vi "LanguageList.vi"(10 "LanguageList":string) -> (0 "Fehler (Ausgang)":errorcluster, 1 "Sprachen Anzahl":i32, 2 "Sprache full":T2 caption="Please select a language:" items=["Deutsch", "English", "Français", "Italiano", "Castellano", "Polski"], 3 "Strings und Werte []":T1, 4 "FullLanguageList":u16[](array[numeric]), 5 "FullLanguageList":string)   [LabVIEW 2015, in "Sprachverwaltung.lvlib"]
doc: "Sprachauswahl für Auswahlfeld nach einer Liste (Indexzahlen getrennt mit Komma) aus der Geasmtsprachliste.\nGibt die Geasmtsprachliste, Anzahl der Sprachen, Indexliste aller Spreachen und die Sprachauswahl zurück.\nRIW 2019-11-29 (Black Friday)s"
uses:
  Sprachverwaltung.lvlib
  Allgemein/Sprachauswahl native.ctl
  <vilib>/Utility/miscctls.llb/LVStringsAndValuesArrayTypeDef_U16.ctl
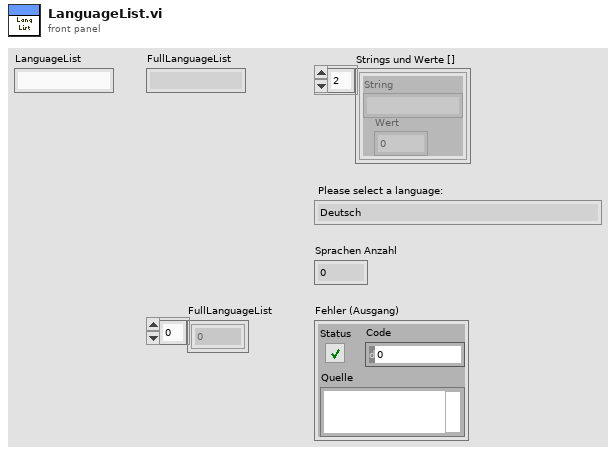
[diagram p1: front panel]
types:
  T1 = typedef "LVStringsAndValuesArrayTypeDef_U16.ctl" = cluster{"String":string, "Value":u16}[]
  T2 = typedef "Sprachverwaltung.lvlib/Sprachauswahl native.ctl" = u16
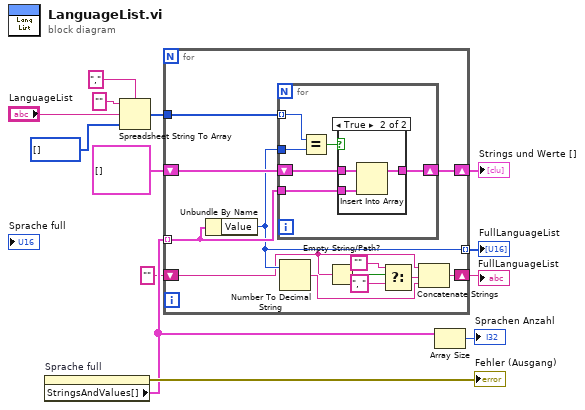
[diagram p0: block diagram]
diagram:
  n1 = property on="Sprache full" class="Ring (strikt)"() -> (error out=→"Fehler (Ausgang)":errorcluster, "StringsAndValues[]"=w5:T1)  [unwired: 2 in, 1 out]
  n2 = Spreadsheet String To Array(delimiter (Tab)="," ("Trennzeichen (Tabulator)"), format string="" ("Format-String"), spreadsheet string="LanguageList", array type (2D Dbl)=u16[] []) -> (array=w11:u16[])
  n3 = for {
    tunnel: w11 -> [w25]
    tunnel: w5 -> [w22] mode=indexing
    shift-right: [w24] -> w6
    shift-left: T1 [] ("Strings und Werte []") -> [w23]
    tunnel: [w21] -> w3 mode=indexing
    shift-right: [w20] -> w2
    shift-left: "" -> [w18]
    n4 = Unbundle By Name(w22) -> ("Value"=w21:u16)
    n5 = for {
      tunnel: w21 -> [w26]
      tunnel: w25 -> [w31] mode=indexing
      tunnel: w22 -> [w29]
      shift-right: [w28] -> w24
      shift-left: w23 -> [w27]
      n6 = Equal?(x=w31, y=w26) -> (x = y?=w30:bool)
      n7 = case shown="True" w30 {
        tunnel: w27 -> [w32 w35]
        tunnel: [w32 w34] -> w28
        tunnel: w29 -> [_ w33]
        frame False {
        }
        frame True {
          n8 = Insert Into Array(array=w35, new element=w33) -> (w34:T1)  [unwired: 1 in]
        }
      }
    }
    n9 = Number To Decimal String(number=w21) -> (decimal integer string=w19:string)  [unwired: 1 in]
    n10 = Empty String/Path?(string/path=w18) -> (empty?=w17:bool)
    n11 = Select(t="", s=w17, f=", " ("String")) -> (s? t:f=w15:string)
    n12 = Concatenate Strings(w18, w15, w19) -> (w20:string)
  }
  "Strings und Werte []" <- w6
  "FullLanguageList" <- w3
  "FullLanguageList" <- w2
  n13 = Array Size(array=w5) -> (size(s)=→"Sprachen Anzahl":i32)
